vi "APC_9056_9049SharedVarPolling.vi"(2 "Number of signals":i32) -> (0 "Number of signals (out)":i32, 1 "9049_CycleAveragedVariables":dbl[](array[numeric]))   [LabVIEW 2020]
doc: "This example demonstrates the procedure required to apply different NI-DAQmx Custom Scales to each virtual channel in a task. A DAQmx Task Property Node (Functions >> NI Measurements >> DAQmx - Data Acquisition >> DAQmx Advanced Task Options) is used to obtain the task's virtual channels. A DAQmx Channel Property Node (Functions >> NI Measurements >> DAQmx - Data Acquisition) is then used to set the custom scale for each virtual channel in the task.\n\nThe \"DAQmx Create Scale\" VI creates a custom scale for each channel in the channel list. *Note, make sure your Minimum and Maximum channel parameters are consistent with the range the scale will create."
panel:
  out "Received signals":i32
  out "9049_raster":string[](array[string])
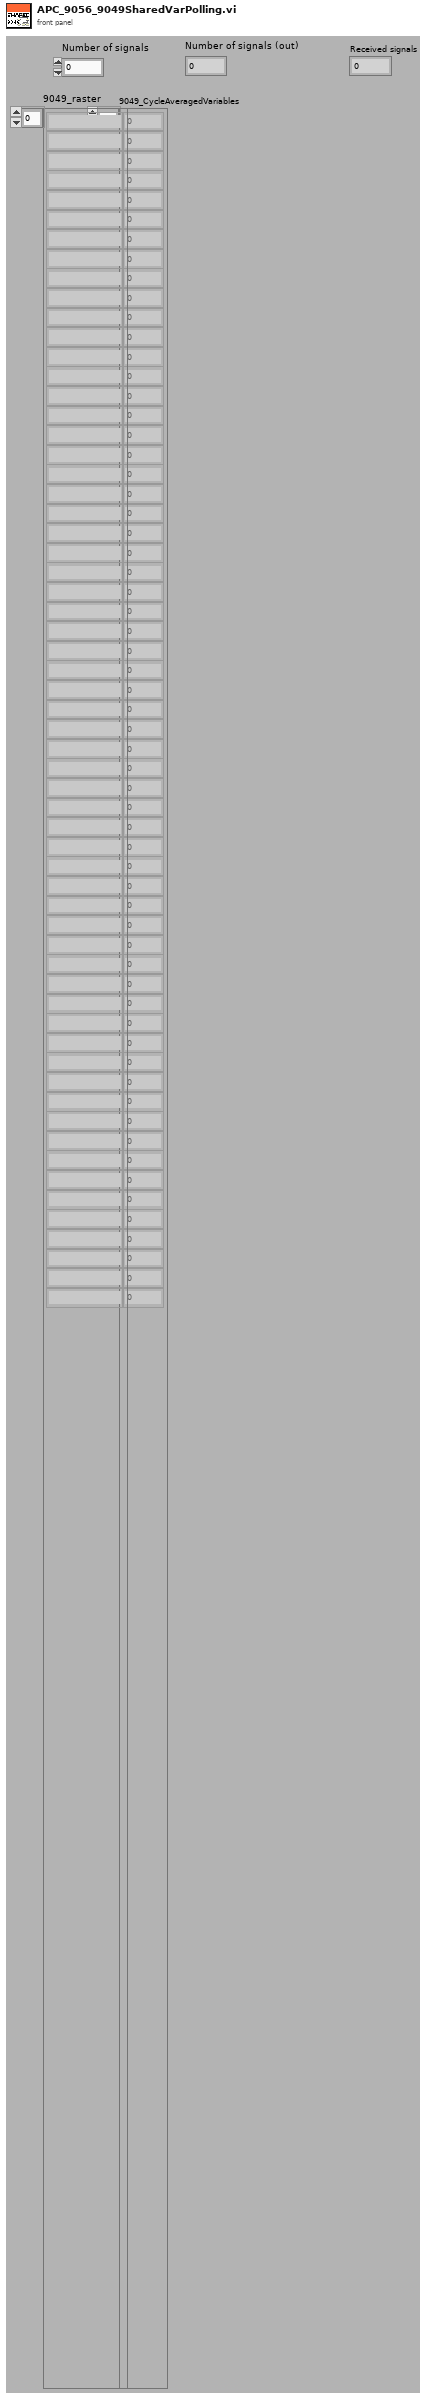
[diagram p1: front panel]
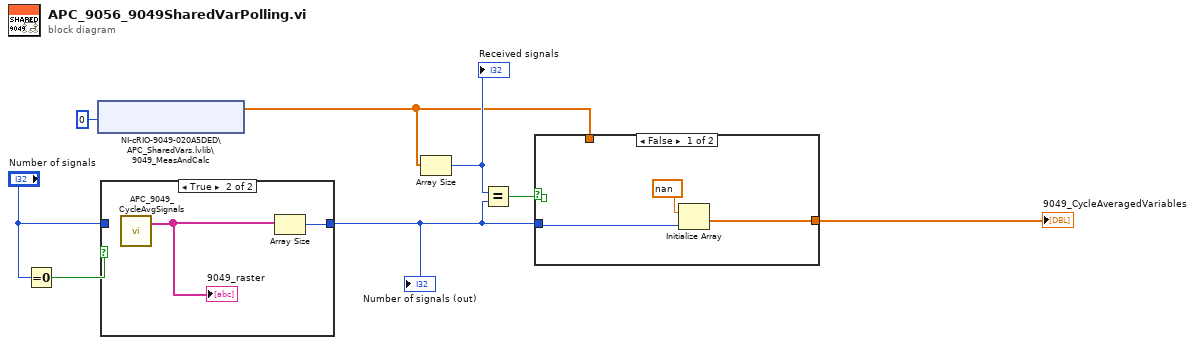
[diagram p0: block diagram]
diagram:
  n1 = Equal To 0?(x="Number of signals") -> (x = 0?=w3:bool)
  n2 = shared-variable "NI-cRIO-9049-020A5DED\\APC_SharedVars.lvlib\\9049_MeasAndCalc"(0 ("ms timeout (0)")) -> (w5:dbl[])  [unwired: 1 in, 2 out]
  n3 = case shown="True" w3 {
    tunnel: [w9 w11] -> w1
    tunnel: "Number of signals" -> [w9 _]
    frame False {
    }
    frame True {
      n4 = call "APC_9049_CycleAvgSignals.vi"() -> ("CRIo9049_CycleAvgSignals"=w10:string[])  [unwired: 3 in]
      "9049_raster" <- w10
      n5 = Array Size(array=w10) -> (size(s)=w11:i32)
    }
  }
  "Number of signals (out)" <- w1
  n6 = Array Size(array=w5) -> (size(s)=w7:i32)
  "Received signals" <- w7
  n7 = Equal?(x=w7, y=w1) -> (x = y?=w6:bool)
  n8 = case shown="False" w6 {
    tunnel: w5 -> [_ w15]
    tunnel: w1 -> [w14 _]
    tunnel: [w12 w15] -> w4
    frame False {
      n9 = Initialize Array(nan ("element"), w14) -> (w12:dbl[])
    }
    frame True {
    }
  }
  "9049_CycleAveragedVariables" <- w4
